vi "After Close.vi"(8 "error in":errorcluster, 9 "State In":variant, 10 "Compiled Settings":variant, 11 "Custom Device API in":refnum<class "Custom Device API.lvclass">) -> (0 "error out":errorcluster, 1 "State Out":variant, 3 "Custom Device API out":refnum<class "Custom Device API.lvclass">)   [LabVIEW 2026, in "SystemMonitor Test Hooks.lvlib"]
uses:
  SystemMonitor Test Hooks.lvlib
  <userlib>/Custom Device Interfaces_v1.lvlibp/CustomDeviceAPI/Custom Device API.lvclass
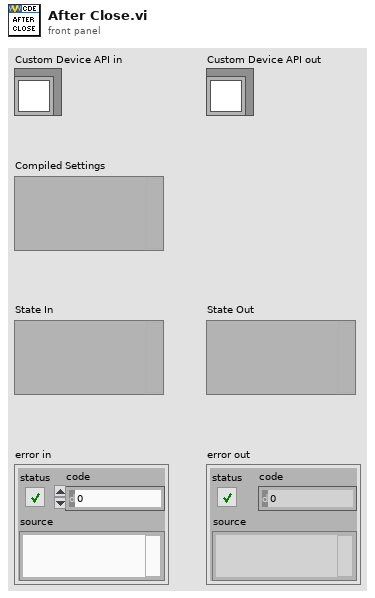
[diagram p1: front panel]
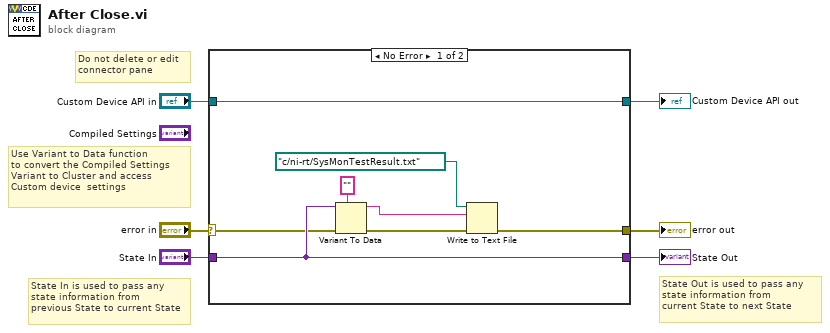
[diagram p0: block diagram]
diagram:
  # "Use Variant to Data function\nto convert the Compiled Settings\nVariant to Cluster and access \nCustom device  settings"
  # "State Out is used to pass any \nstate information from\ncurrent State to next State"
  # "State In is used to pass any \nstate information from\nprevious State to current State"
  # "Do not delete or edit \nconnector pane"
  n1 = case shown="No Error" "error in" {
    selector: "error in" -> [w9 w16]
    tunnel: [w7 w16] -> w5
    tunnel: "Custom Device API in" -> [w14 w17]
    tunnel: [w14 w17] -> w3
    tunnel: "State In" -> [w13 w15]
    tunnel: [w13 w15] -> w1
    frame No Error {
      n2 = Variant To Data(error in=w9, type="", Variant=w13) -> (data=w11:string, error out=w8:errorcluster)
      n3 = Write to Text File(file (use dialog)=path "c:/ni-rt/SysMonTestResult.txt", text=w11, error in=w8) -> (error out=w7:errorcluster)  [unwired: 1 in, 2 out]
    }
    frame Error {
    }
  }
  "Custom Device API out" <- w3
  "error out" <- w5
  "State Out" <- w1
